vi "2019-05-013_SequenceStructure_02.vi"() -> ()   [LabVIEW 2018]
panel:
  out "웨이브폼 차트":dbl(graph)
  out "x-y":u32
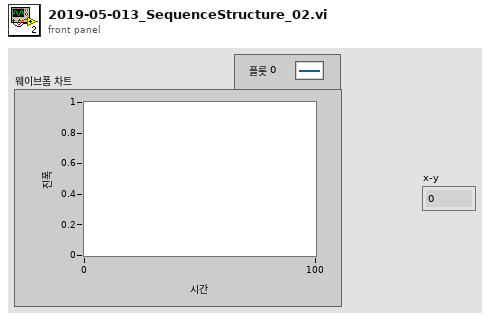
[diagram p1: front panel]
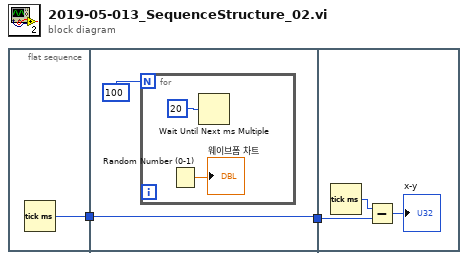
[diagram p0: block diagram]
diagram:
  n1 = flat-sequence {
    tunnel: [w3] -> w1
    tunnel: [w4] -> w2
    tunnel: w1 -> [w4]
    tunnel: w2 -> [w9]
    frame #0 {
      n2 = Tick Count (ms)() -> (millisecond timer value=w3:u32)
    }
    frame #1 {
      n3 = for {
        N: 100 -> [_]
        n4 = Random Number (0-1)() -> (number: 0 to 1=→"웨이브폼 차트":dbl)
        n5 = Wait Until Next ms Multiple(millisecond multiple=20) -> ()  [unwired: 1 out]
      }
    }
    frame #2 {
      n6 = Tick Count (ms)() -> (millisecond timer value=w10:u32)
      n7 = Subtract(x=w10, y=w9) -> (x-y=→"x-y":u32)
    }
  }
